vi "Do Core.vi"(8 "error in":errorcluster, 9 "Actor in":refnum<class "Actor.lvclass">, 11 "DS Reply Msg in":refnum<class "Reply Msg DataSocket AE Msg.lvclass">) -> (0 "error out":errorcluster, 1 "Actor out":refnum<class "Actor.lvclass">, 2 "Reply":variant)   [LabVIEW 2023, in "Target Reply Time Test Actor.lvlib" / "Reply Msg DataSocket AE Msg.lvclass"]
uses:
  <vilib>/ActorFramework/Actor/Actor.lvclass
  Reply Msg DataSocket AE Msg.lvclass
  Reply Msg DataSocket AE Msg.lvclass/Reply Msg DataSocket AE Msg.ctl
  Target Reply Time Test Actor/Target Reply Time Test Actor.lvclass
  7ce3314c-3766-4d96-9999-254d5ed4d181.vi
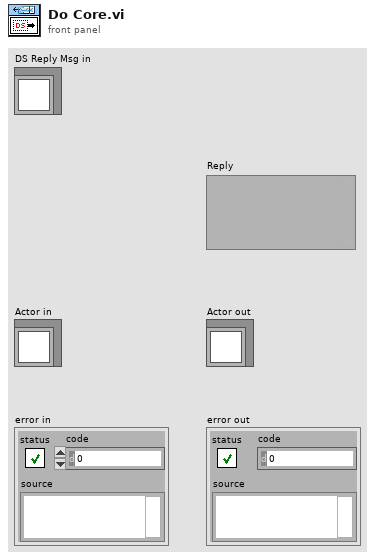
[diagram p1: front panel]
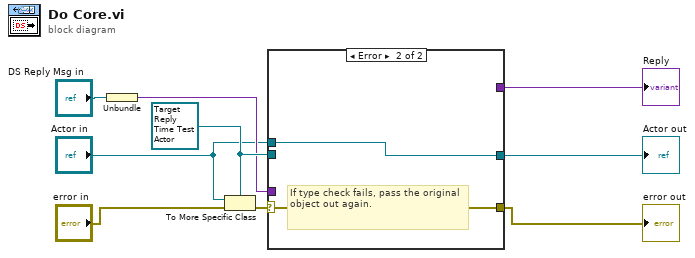
[diagram p0: block diagram]
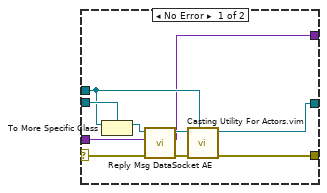
[diagram p2: hidden frame]
diagram:
  w8 = refnum<class "Target Reply Time Test Actor.lvclass"> refnum ("Actor in")
  n1 = Unbundle("DS Reply Msg in") -> (w7:variant)
  n2 = To More Specific Class(target class=w8, reference="Actor in", error in="error in") -> (error out=w9:errorcluster)  [unwired: 1 out]
  n3 = case shown="Error" w9 {
    selector: w9 -> [w19 w21]
    tunnel: [w13 w21] -> w5
    tunnel: [w14 w20] -> w4
    tunnel: "Actor in" -> [w16 w20]
    tunnel: w8 -> [w17 _]
    tunnel: w7 -> [w11 _]
    tunnel: [w10 _] -> w1
    frame No Error {
      n4 = To More Specific Class(target class=w17, reference=w16) -> (specific class reference=w18:refnum<class "Target Reply Time Test Actor.lvclass">)  [unwired: 1 in, 1 out]
      n5 = call-dynamic "Reply Msg DataSocket AE.vi"("error in (no error)"=w19, "Input"=w11, "Target Reply Time Test Actor in"=w18) -> ("error out"=w12:errorcluster, "Reply"=w10:variant, "Target Reply Time Test Actor out"=w15:refnum<class "Target Reply Time Test Actor.lvclass">)  [unwired: 6 in]
      n6 = call "Casting Utility For Actors.vim"("type"=w16, "error in (no error)"=w12, "Actor in"=w15) -> ("error out"=w13:errorcluster, "Actor out"=w14:refnum<class "Actor.lvclass">)  [unwired: 7 in]
    }
    frame Error {
      # "If type check fails, pass the original object out again."
    }
  }
  "error out" <- w5
  "Actor out" <- w4
  "Reply" <- w1
